vi "ZBX DB Set Gain.vi"(4 "response in":T1, 7 "ATR state":T3, 8 "rx gain valid":bool, 9 "rx gain":u32, 10 "tx gain valid":bool, 11 "tx gain":u32) -> (5 "request out":T2)   [LabVIEW 2023]
uses:
  <instrlib>/niUSRP/Reference FPGA/ZBX Control/Antenna.ctl
  <instrlib>/niUSRP/Reference FPGA/ZBX Control/ATR state.ctl
  <instrlib>/niUSRP/Reference FPGA/ZBX Control/ZBX IO Request.ctl
  <instrlib>/niUSRP/Reference FPGA/ZBX Control/ZBX IO Response.ctl
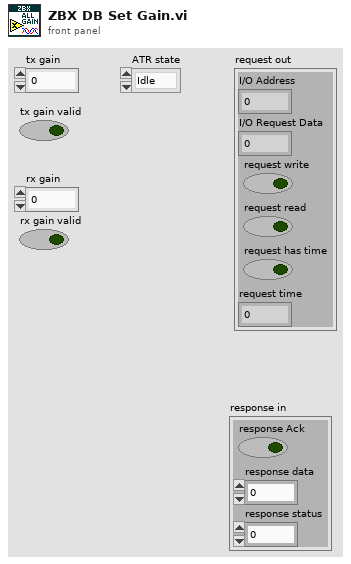
[diagram p1: front panel]
types:
  T1 = typedef "ZBX IO Response.ctl" = cluster{"response Ack":bool, "response data":u32, "response status":fxp<+,2,2>}
  T2 = typedef "ZBX IO Request.ctl" = cluster{"I/O Address":fxp<+,20,20>, "I/O Request Data":u32, "request write":bool, "request read":bool, "request has time":bool, "request time":u64}
  T3 = typedef "ATR state.ctl" = enum8{"Idle", "RX", "TX", "TRX"}
  T4 = typedef "Antenna.ctl" = enum8{"tx/0", "tx/1", "rx/0", "rx/1"}
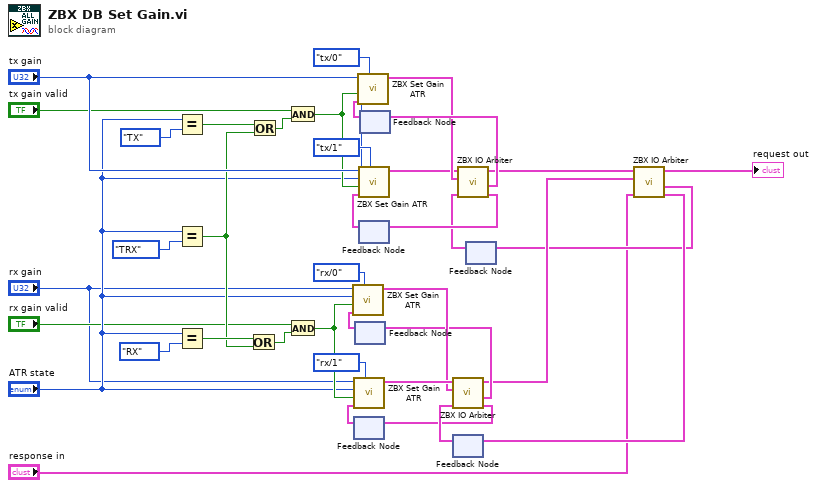
[diagram p0: block diagram]
diagram:
  n1 = Equal?(x="ATR state", y=ATR_state."TX") -> (x = y?=w13:bool)
  n2 = Equal?(x="ATR state", y=ATR_state."TRX") -> (x = y?=w11:bool)
  n3 = Equal?(x="ATR state", y=ATR_state."RX") -> (x = y?=w12:bool)
  n4 = Or(x=w12, y=w11) -> (x .or. y?=w3:bool)
  n5 = Or(x=w13, y=w11) -> (x .or. y?=w10:bool)
  n6 = And(x="tx gain valid", y=w10) -> (x .and. y?=w9:bool)
  n7 = And(x="rx gain valid", y=w3) -> (x .and. y?=w7:bool)
  n8 = feedback #1() -> (w36:T1)  [unwired: 1 in]
  n9 = call <instrlib>:"ZBX Set Gain ATR.vi"("channel"=Antenna."rx/1" ("Antenna"), "response"=w36, "input valid"=w7, "ATR state"="ATR state", "gain"="rx gain") -> ("request"=w37:T2)  [unwired: 6 in]
  n10 = feedback #2() -> (w31:T1)  [unwired: 1 in]
  n11 = call <instrlib>:"ZBX Set Gain ATR.vi"("channel"=Antenna."rx/0" ("Antenna"), "response"=w31, "input valid"=w7, "ATR state"="ATR state", "gain"="rx gain") -> ("request"=w34:T2)  [unwired: 6 in]
  n12 = feedback #3() -> (w23:T1)  [unwired: 1 in]
  n13 = call <instrlib>:"ZBX Set Gain ATR.vi"("channel"=Antenna."tx/1" ("Antenna"), "response"=w23, "input valid"=w9, "ATR state"="ATR state", "gain"="tx gain") -> ("request"=w22:T2)  [unwired: 6 in]
  n14 = feedback #4() -> (w28:T1)  [unwired: 1 in]
  n15 = call <instrlib>:"ZBX Set Gain ATR.vi"("channel"=Antenna."tx/0" ("Antenna"), "response"=w28, "input valid"=w9, "ATR state"="ATR state", "gain"="tx gain") -> ("request"=w25:T2)  [unwired: 6 in]
  n16 = feedback #5() -> (w38:T1)  [unwired: 1 in]
  n17 = call <instrlib>:"ZBX IO Arbiter.vi"("response"=w38, "request 2"=w34, "request 1"=w37) -> ("response 2"=w33:T1, "response1"=w32:T1, "request out"=w21:T2)  [unwired: 5 in, 1 out]
  n18 = feedback-in #1(w33) -> ()
  n19 = feedback-in #2(w32) -> ()
  n20 = feedback #6() -> (w17:T1)  [unwired: 1 in]
  n21 = call <instrlib>:"ZBX IO Arbiter.vi"("response"=w17, "request 2"=w25, "request 1"=w22) -> ("response 2"=w26:T1, "response1"=w27:T1, "request out"=w20:T2)  [unwired: 5 in, 1 out]
  n22 = feedback-in #3(w26) -> ()
  n23 = feedback-in #4(w27) -> ()
  n24 = call <instrlib>:"ZBX IO Arbiter.vi"("response"="response in", "request 2"=w21, "request 1"=w20) -> ("response 2"=w19:T1, "response1"=w18:T1, "request out"=→"request out":T2)  [unwired: 5 in, 1 out]
  n25 = feedback-in #5(w19) -> ()
  n26 = feedback-in #6(w18) -> ()
